vi "write_timing_array.vi"(4 "error in":errorcluster, 5 "delay array":dbl[](array[numeric]), 7 "VISA resource in":refnum<visa-resource-name>) -> (0 "error out 2":errorcluster, 3 "VISA resource out":refnum<visa-resource-name>)   [LabVIEW 2012]
doc: "Reads all delay values stored in the DG645 and returns them in an array, from t0 to H.\nSee DG645 documentation for mor info."
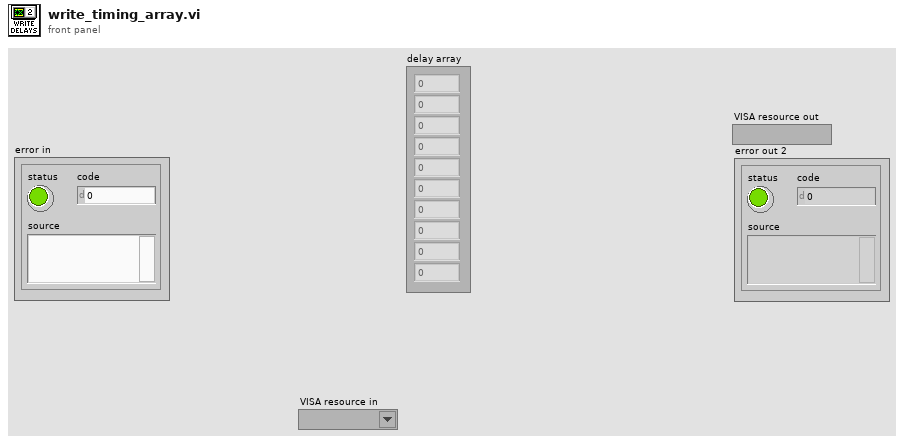
[diagram p1: front panel]
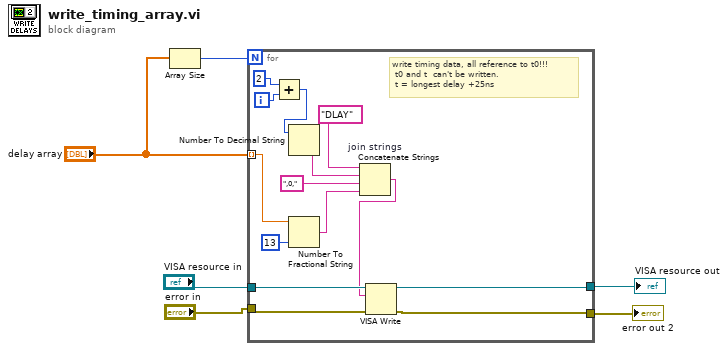
[diagram p0: block diagram]
diagram:
  n1 = Array Size(array="delay array") -> (size(s)=w1:i32)
  n2 = for {
    N: w1 -> [_]
    tunnel: "error in" -> [w18]
    tunnel: [w19] -> w3
    tunnel: "VISA resource in" -> [w15]
    tunnel: [w20] -> w4
    tunnel: "delay array" -> [w10] mode=indexing
    i -> [w13]
    # "write timing data, all reference to t0!!!\n t0 and t  can't be written.\n t = longest delay +25ns"
    n3 = Add(x=2, y=w13) -> (x+y=w8:i32)
    n4 = Number To Decimal String(number=w8) -> (decimal integer string=w16:string)  [unwired: 1 in]
    n5 = Number To Fractional String(number=w10, precision (6)=i16 13) -> (F-format string=w12:string)  [unwired: 2 in]
    n6 = Concatenate Strings "join strings"("DLAY" ("string"), w16, ",0," ("string"), w12) -> (w11:string)
    n7 = VISA Write(VISA resource name=w15, write buffer=w11, error in (no error)=w18) -> (VISA resource name out=w20:refnum<visa-resource-name>, error out=w19:errorcluster)  [unwired: 1 out]
  }
  "VISA resource out" <- w4
  "error out 2" <- w3
